vi "WriteXmlFileProperties.vi"(2 "error in":errorcluster, 3 "NameFileAndType":string, 4 "Parameters":variant) -> (0 "error out":errorcluster, 1 "PathXMLFile":path)   [LabVIEW 2010]
uses:
  <vilib>/Utility/xml.llb/Write to XML File(string).vi
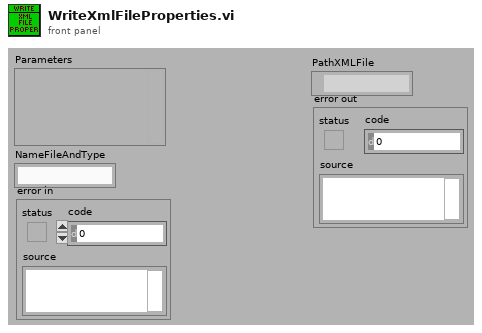
[diagram p1: front panel]
types:
  T1 = enum16{"open", "replace", "create", "open or create", "replace or create", "replace or create with confirmation"}
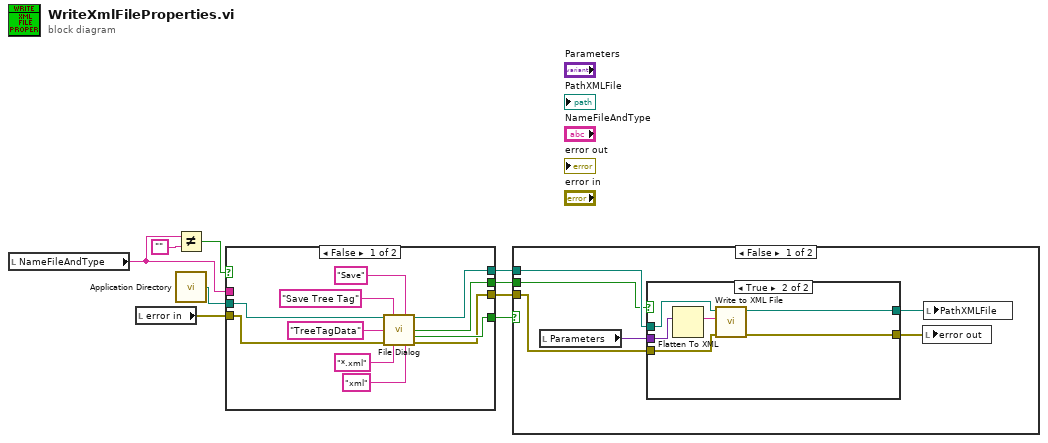
[diagram p0: block diagram]
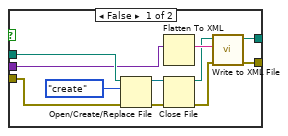
[diagram p2: hidden frame]
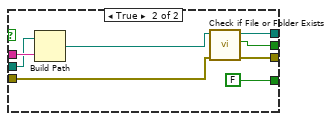
[diagram p4: hidden frame]
diagram:
  n1 = local read "NameFileAndType"() -> (w3:string)
  n2 = local read "error in"() -> (w6:errorcluster)
  n3 = Not Equal?(x=w3, y="") -> (x != y?=w2:bool)
  n4 = call <vilib>:"Application Directory.vi"() -> ("Application Directory"=w5:path)
  n5 = case shown="False" w2 {
    tunnel: [w10 w27] -> w9
    tunnel: w3 -> [_ w26]
    tunnel: [w12 w25] -> w8
    tunnel: [w11 w24] -> w7
    tunnel: w6 -> [w19 w23]
    tunnel: w5 -> [w20 w22]
    tunnel: [w13 FALSE ("cancelled")] -> w1
    frame False {
      n6 = call "File Dialog"("start path"=w20, "prompt"="Save Tree Tag", "button label"="Save", "default name"="TreeTagData", "error in"=w19, "pattern (all files)"="*.xml", "pattern label"="xml") -> ("selected path"=w10:path, "exists"=w12:bool, "cancelled"=w13:bool, "error out"=w11:errorcluster)  [unwired: 5 in]
    }
    frame True {
      n7 = Build Path(base path=w22, name or relative path=w26) -> (appended path=w28:path)
      n8 = call <vilib>:"Check if File or Folder Exists.vi"("error in (no error)"=w23, "path"=w28) -> ("error out"=w24:errorcluster, "file or folder exists?"=w25:bool, "dup path"=w27:path)  [unwired: 7 in]
    }
  }
  n9 = case shown="False" w1 {
    tunnel: w9 -> [w34 _]
    tunnel: w8 -> [w30 _]
    tunnel: w7 -> [w29 _]
    frame False {
      n10 = local read "Parameters"() -> (w33:variant)
      n11 = case shown="True" w30 {
        tunnel: w34 -> [w39 w50]
        tunnel: w33 -> [w38 w49]
        tunnel: [w37 w48] -> w31
        tunnel: [w36 w47] -> w32
        tunnel: w29 -> [w35 w46]
        frame False {
          n12 = Open/Create/Replace File(file path (use dialog)=w39, error in=w35, operation (0:open)=T1."create") -> (refnum out=w43:refnum<file>, error out=w42:errorcluster)  [unwired: 3 in, 1 out]
          n13 = Flatten To XML(anything=w38) -> (xml string=w44:string)
          n14 = Close File(refnum=w43, error in=w42) -> (path=w41:path, error out=w40:errorcluster)
          n15 = call-poly <vilib>:"Write to XML File.vi"("error in (no error)"=w40, "XML Input"=w44, "XML File Path"=w41) -> ("error out"=w37:errorcluster, "XML File Path(duplicate)"=w36:path)  [unwired: 6 in, 1 out]
        }
        frame True {
          n16 = Flatten To XML(anything=w49) -> (xml string=w51:string)
          n17 = call-poly <vilib>:"Write to XML File.vi"("error in (no error)"=w46, "XML Input"=w51, "XML File Path"=w50) -> ("error out"=w48:errorcluster, "XML File Path(duplicate)"=w47:path)  [unwired: 6 in, 1 out]
        }
      }
      n18 = local write "error out"(w31) -> ()
      n19 = local write "PathXMLFile"(w32) -> ()
    }
    frame True {
    }
  }
